vi "Codes Filtering.vi"(10 "searched objects":string[](array[string]), 11 "scope error codes":i32[](array[numeric])) -> (3 "found codes indices":i32[](array[numeric]))   [LabVIEW 2017]
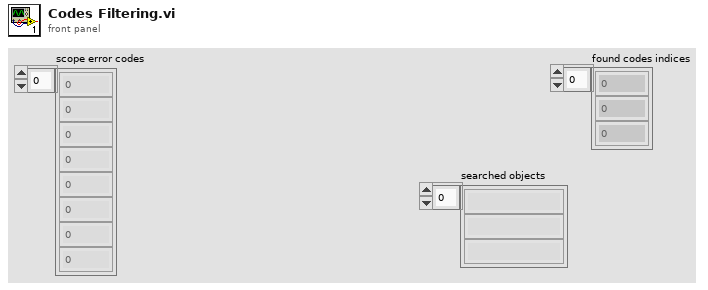
[diagram p1: front panel]
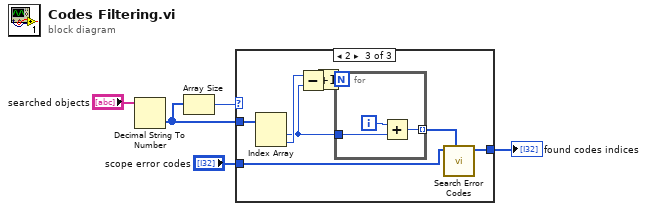
[diagram p0: block diagram]
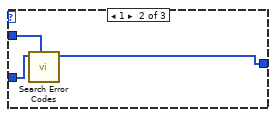
[diagram p3: hidden frame]
diagram:
  n1 = Decimal String To Number(string="searched objects") -> (number=w2:i32[])  [unwired: 2 in, 1 out]
  n2 = Array Size(array=w2) -> (size(s)=w5:i32)
  n3 = case shown="2" w5 {
    tunnel: w2 -> [_ w8 w13]
    tunnel: "scope error codes" -> [_ w7 w12]
    tunnel: [_ w6 w10] -> w1
    frame Default {
    }
    frame 1 {
      n4 = call "Search Error Codes.vi"("searched objects"=w8, "scope error codes"=w7) -> ("found codes indices"=w6:i32[])  [unwired: 9 in]
    }
    frame 2 {
      n5 = Index Array(array=w13) -> (element #1=w15:i32, element #2=w16:i32)  [unwired: 2 in]
      n6 = Subtract(x=w16, y=w15) -> (x-y=w14:i32)
      n7 = Increment(x=w14) -> (x+1=w9:i32)
      n8 = for {
        N: w9 -> [_]
        tunnel: w15 -> [w18]
        tunnel: [w17] -> w11 mode=indexing
        i -> [w19]
        n9 = Add(x=w19, y=w18) -> (x+y=w17:i32)
      }
      n10 = call "Search Error Codes.vi"("searched objects"=w11, "scope error codes"=w12) -> ("found codes indices"=w10:i32[])  [unwired: 9 in]
    }
  }
  "found codes indices" <- w1
